vi "ToogleLifeBitFromLabview.vi"(11 "input bool array":bool[](array[boolean])) -> (3 "output bool array":bool[](array[boolean]))   [LabVIEW 2020]
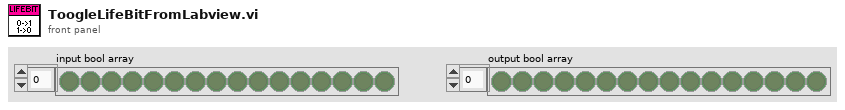
[diagram p1: front panel]
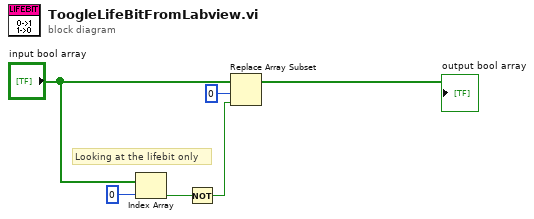
[diagram p0: block diagram]
diagram:
  # "Looking at the lifebit only"
  n1 = Index Array(array="input bool array", index=0) -> (element=w6:bool)
  n2 = Not(x=w6) -> (.not. x?=w4:bool)
  n3 = Replace Array Subset(array="input bool array", new element=w4, index=0) -> (→"output bool array":bool[])
